vi "get Port Name.vi"(8 "error in (no error)":errorcluster, 11 "port_num":i32) -> (0 "error out":errorcluster, 3 "function return":string)   [LabVIEW 2018, in "labview.lvlib"]
doc: "WINDECLSPEC char *getPortName (int port_num);"
uses:
  labview.lvlib
  dxl_x86_c.dll
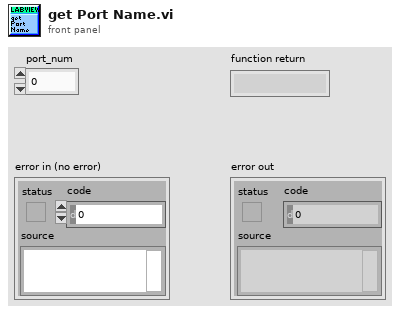
[diagram p1: front panel]
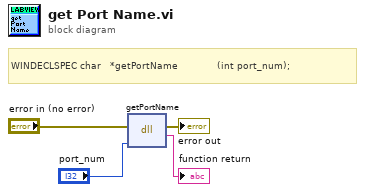
[diagram p0: block diagram]
diagram:
  # "WINDECLSPEC char   *getPortName             (int port_num);"
  n1 = dll-call lib="C:/Users/joaos/OneDrive/Documents/[PhD]/Project Omnidirectional Vehicle/Vanes/LabView_code/joaoandthethreestands/DynamixelSDK-3.7.31/labview/new_compilation/dxl_x86_c.*" fn="getPortName"(error in="error in (no error)", "port_num"="port_num") -> (error out=→"error out":errorcluster, →"function return":string)  [unwired: 3 in, 1 out]
